vi "Language Write.vi"(4 "error in (no error)":errorcluster, 5 "Value":T1, 6 "Container State":T3, 7 "Display State In":T2) -> (0 "error out":errorcluster, 3 "Display State Out":T2)   [LabVIEW 2011, in "Calendar XControl.xctl"]
uses:
  Calendar XControl.xctl
  <vilib>/_xctls/Container State.ctl
  State 2.ctl
  Language selection.ctl
  <vilib>/_xctls/XControlSupport.lvlib
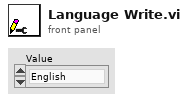
[diagram p1: front panel]
types:
  T1 = typedef "Calendar XControl.xctl/Language selection.ctl" = enum16{"English", "Français", "Español", "Deutsche", "Italiano", "Svenska", "Portugese"}
  T2 = typedef "Calendar XControl.xctl/State 2.ctl" = cluster{"Language selection":T1, "Time Stamp":timestamp}
  T3 = typedef "XControlSupport.lvlib/Container State.ctl" = cluster{"Indicator?":bool, "Run Mode?":bool, " Refnum":refnum<vi>}
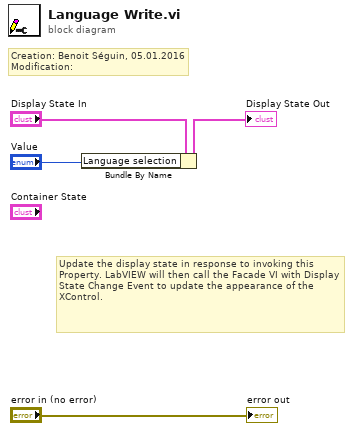
[diagram p0: block diagram]
diagram:
  # "Creation: Benoit Séguin, 05.01.2016\nModification:"
  # "Update the display state in response to invoking this Property. LabVIEW will then call the Facade VI with Display State Change Event to update the appearance of the XControl."
  n1 = Bundle By Name(cluster="Display State In", "Language selection"="Value") -> (→"Display State Out":T2)
  "error out" <- "error in (no error)"
